vi "OA Get Float.vi"(8 "error in (no error)":errorcluster, 9 "fFloatValue":sgl, 10 "pcModeParam":string, 11 "pcModeName":string) -> (0 "error out":errorcluster, 1 "fFloatValue out":sgl, 3 "function return":u32)   [LabVIEW 2014, in "atmcd32d.lvlib"]
doc: "unsigned int WINAPI OA_GetFloat(const char * const pcModeName, const char * const pcModeParam, float * fFloatValue);"
uses:
  atmcd32d.lvlib
  atmcd32d.dll
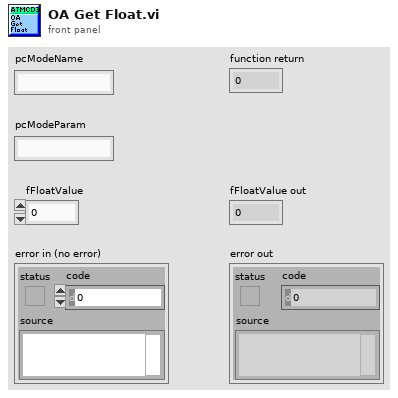
[diagram p1: front panel]
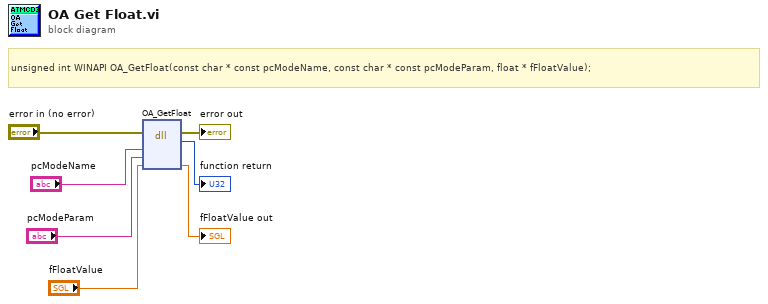
[diagram p0: block diagram]
diagram:
  # "unsigned int WINAPI OA_GetFloat(const char * const pcModeName, const char * const pcModeParam, float * fFloatValue);"
  n1 = dll-call lib="C:/Users/Bakir/Documents/Lambda2-Testing/lib/Andorlib/atmcd32d.*" fn="OA_GetFloat"(error in="error in (no error)", "pcModeName"="pcModeName", "pcModeParam"="pcModeParam", "fFloatValue"="fFloatValue") -> (error out=→"error out":errorcluster, →"function return":u32, "fFloatValue"=→"fFloatValue out":sgl)  [unwired: 4 in, 1 out]
